vi "SigCon.vi"(11 "data":dynamicdata(waveform)) -> (3 "data 2":dynamicdata(waveform) caption="data")   [LabVIEW 2020]
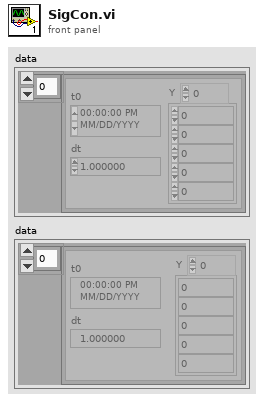
[diagram p1: front panel]
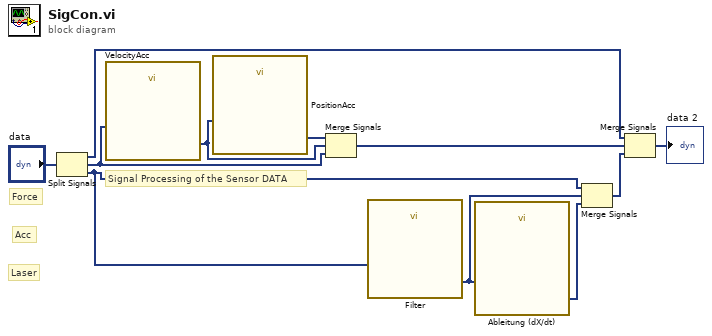
[diagram p0: block diagram]
diagram:
  # "Laser"
  # "Acc"
  # "Force"
  # "Signal Processing of the Sensor DATA"
  n1 = Split Signals("data") -> (w1:dynamicdata, w2:dynamicdata, w3:dynamicdata)  [unwired: 3 in]
  n2 = call "VelocityAcc"("Signals"=w2) -> ("Result"=w9:dynamicdata)  [unwired: 5 in, 1 out]
  n3 = call "PositionAcc"("Signals"=w9) -> ("Result"=w10:dynamicdata)  [unwired: 5 in, 1 out]
  n4 = Merge Signals(w10, w9, w2) -> (w6:dynamicdata)
  n5 = call "Filter"("Signal"=w3) -> ("Filtered Signal"=w4:dynamicdata)  [unwired: 9 in, 1 out]
  n6 = call "Ableitung (dX/dt)"("Signals"=w4) -> ("Result"=w11:dynamicdata)  [unwired: 5 in, 1 out]
  n7 = Merge Signals(w3, w4, w11) -> (w7:dynamicdata)
  n8 = Merge Signals(w1, w6, w7) -> (→"data 2":dynamicdata)
